vi "DO sensor decode.vi"(9 "DO input":string) -> (1 "DO output":dbl[](array[numeric]), 3 "DO output string":string[](array[string]))   [LabVIEW 2021]
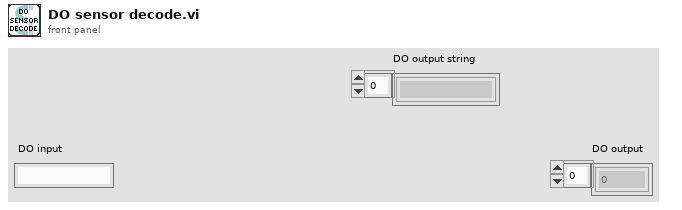
[diagram p1: front panel]
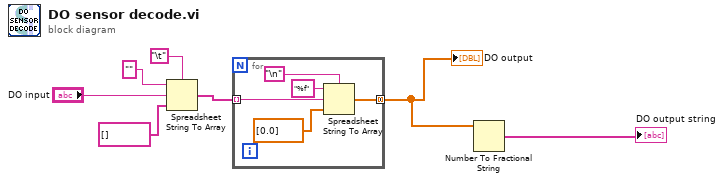
[diagram p0: block diagram]
diagram:
  n1 = Spreadsheet String To Array(delimiter (Tab)="\t", format string="", spreadsheet string="DO input", array type (2D Dbl)=string[] []) -> (array=w4:string[])
  n2 = for {
    tunnel: w4 -> [w11] mode=indexing
    tunnel: [w9] -> w2 mode=concatenating
    n3 = Spreadsheet String To Array(delimiter (Tab)="\n", format string="%f", spreadsheet string=w11, array type (2D Dbl)=dbl[] [0.0]) -> (array=w9:dbl[])
  }
  "DO output" <- w2
  n4 = Number To Fractional String(number=w2) -> (F-format string=→"DO output string":string[])  [unwired: 3 in]
